vi "CalcRotationAngles.vi"(7 "ZAxis":dbl, 9 "XAxis":dbl, 11 "YAxis":dbl) -> (4 "Angles":dbl[](array[numeric]), 6 "Speeds":dbl[](array[numeric]))   [LabVIEW 2018]
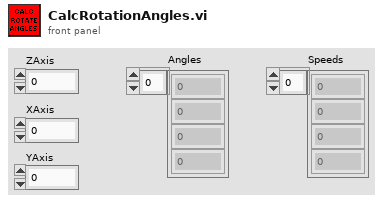
[diagram p1: front panel]
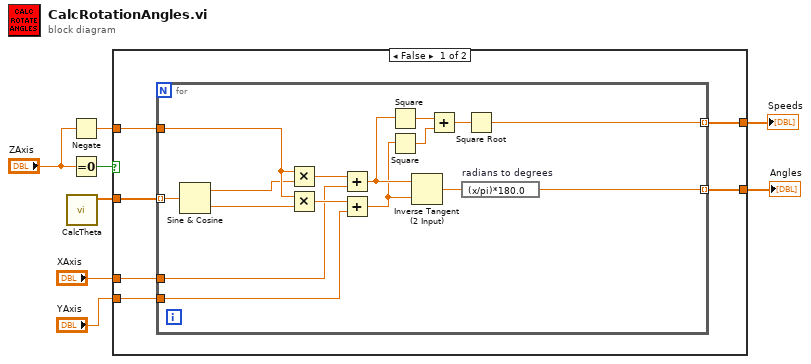
[diagram p0: block diagram]
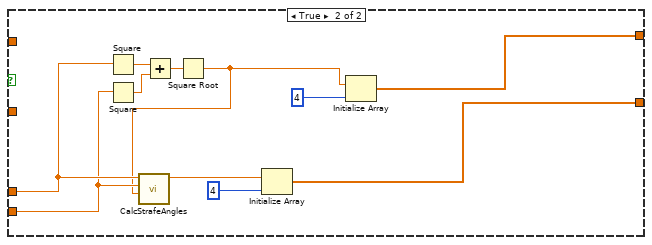
[diagram p2: hidden frame]
diagram:
  n1 = call "CalcTheta.vi"() -> ("ThetaValues"=w5:dbl[])  [unwired: 11 in]
  n2 = Negate(x="ZAxis") -> (-x=w1:dbl)
  n3 = Equal To 0?(x="ZAxis") -> (x = 0?=w7:bool)
  n4 = case shown="False" w7 {
    tunnel: [w14 w38] -> w4
    tunnel: [w13 w39] -> w8
    tunnel: w5 -> [w12 _]
    tunnel: "XAxis" -> [w11 w33]
    tunnel: "YAxis" -> [w10 w32]
    tunnel: w1 -> [w9 _]
    frame False {
      n5 = for {
        tunnel: w12 -> [w30] mode=indexing
        tunnel: w9 -> [w29]
        tunnel: w11 -> [w17]
        tunnel: w10 -> [w16]
        tunnel: [w19] -> w14 mode=indexing
        tunnel: [w20] -> w13 mode=indexing
        n6 = Sine & Cosine(0:w30) -> (1:w15:dbl, 2:w18:dbl)
        n7 = Multiply(x=w29, y=w15) -> (x*y=w27:dbl)
        n8 = Multiply(x=w29, y=w18) -> (x*y=w28:dbl)
        n9 = Add(x=w27, y=w17) -> (x+y=w25:dbl)
        n10 = Add(x=w28, y=w16) -> (x+y=w24:dbl)
        n11 = Square(x=w25) -> (x^2=w23:dbl)
        n12 = Square(x=w24) -> (x^2=w22:dbl)
        n13 = Inverse Tangent (2 Input)(1:w24, 2:w25) -> (0:w26:dbl)
        n14 = Add(x=w23, y=w22) -> (x+y=w21:dbl)
        n15 = expression code="(x/pi)*180.0" "radians to degrees"(w26) -> (w19:dbl)
        n16 = Square Root(x=w21) -> (sqrt(x)=w20:dbl)
      }
    }
    frame True {
      n17 = Square(x=w33) -> (x^2=w37:dbl)
      n18 = Square(x=w32) -> (x^2=w36:dbl)
      n19 = Add(x=w37, y=w36) -> (x+y=w35:dbl)
      n20 = Square Root(x=w35) -> (sqrt(x)=w31:dbl)
      n21 = call "CalcStrafeAngles.vi"("Speed"=w31, "Y"=w32, "X"=w33) -> ("StrafeAngle"=w34:dbl)  [unwired: 8 in]
      n22 = Initialize Array(w34, 4 ("dimension size")) -> (w38:dbl[])
      n23 = Initialize Array(w31, 4 ("dimension size")) -> (w39:dbl[])
    }
  }
  "Angles" <- w4
  "Speeds" <- w8
